vi "Construct Contour SPINE Array (SubVI).vi"(11 "DATA Cluster":T1) -> (0 "Larvae Valid?":bool[](array[boolean]), 1 "Larvae ID":u32[](array[numeric]), 2 "SPINE":cluster{"Array":dbl[], "Array":dbl[]}[](array[cluster]), 3 "Contour":cluster{"Array":i32[], "Array":i32[]}[](array[cluster]), 4 "Frame Valid?":bool)   [LabVIEW 2020]
uses:
  Controls (HOST)/Data to Disk Bundle.ctl
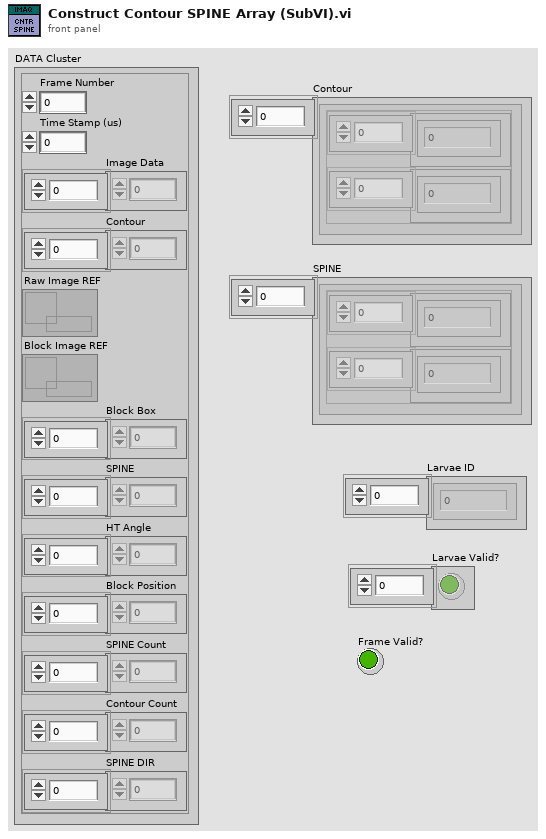
[diagram p1: front panel]
types:
  T1 = typedef "Data to Disk Bundle.ctl" = cluster{"Frame Number":u64, "Time Stamp (us)":u64, "Image Data":u64[], "Contour":u32[], "Raw Image REF":refnum<data-value>, "Block Image REF":refnum<data-value>, "Block Box":u64[], "SPINE":u32[], "HT Angle":u64[], "Block Position":u64[], "SPINE Count":u32[], "Contour Count":u32[], "SPINE DIR":u8[]}
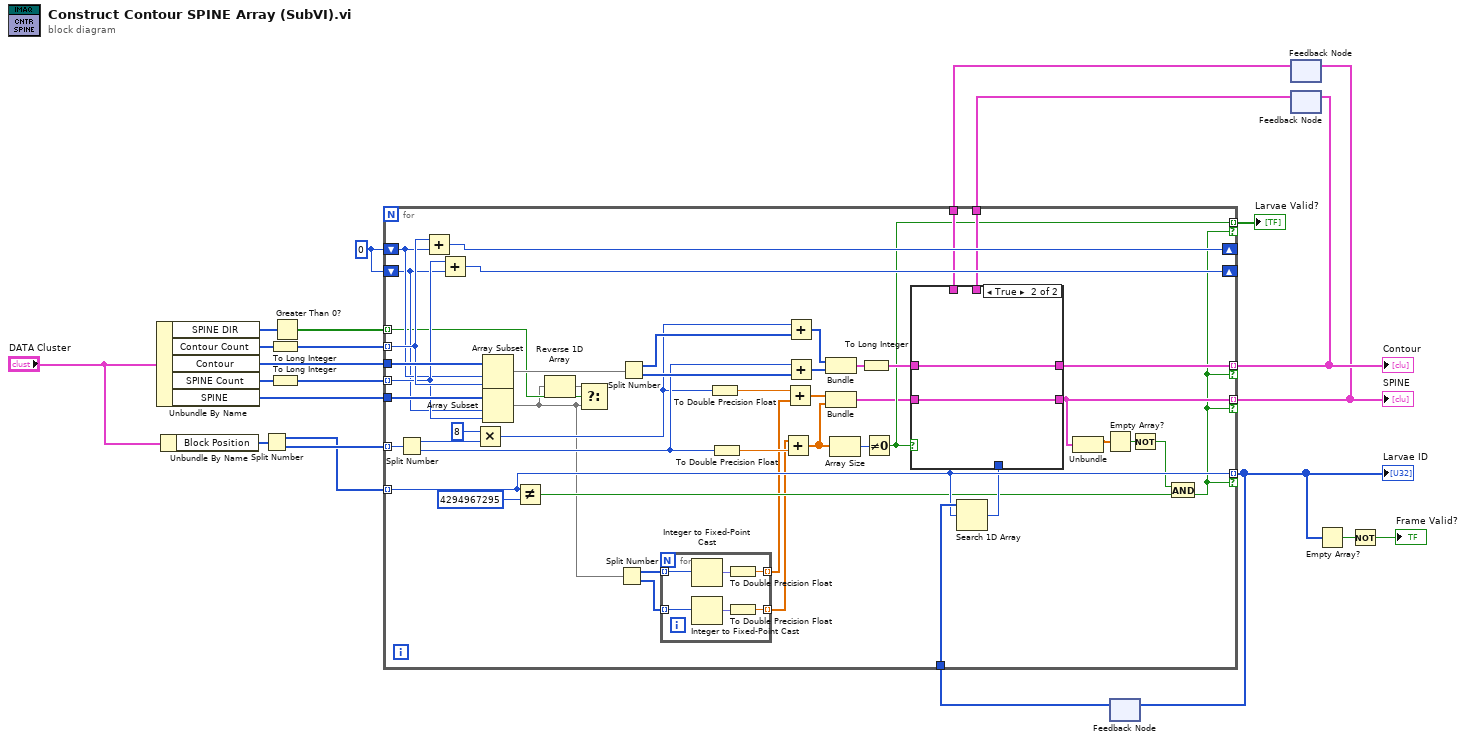
[diagram p0: block diagram]
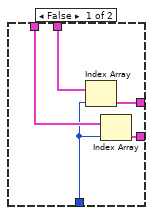
[diagram p2: hidden frame]
diagram:
  w20 = 0 ("Numeric Control")
  n1 = Unbundle By Name("DATA Cluster") -> ("SPINE DIR"=w12:u8[], "Contour Count"=w16:u32[], "Contour"=w17:u32[], "SPINE Count"=w18:u32[], "SPINE"=w19:u32[])
  n2 = Unbundle By Name("DATA Cluster") -> ("Block Position"=w14:u64[])
  n3 = Split Number(x=w14) -> (hi(x)=w10:u32[], lo(x)=w13:u32[])
  n4 = To Long Integer(number=w16) -> (32bit integer=w21:i32[])
  n5 = To Long Integer(number=w18) -> (32bit integer=w22:i32[])
  n6 = Greater Than 0?(x=w12) -> (x > 0?=w11:bool[])
  n7 = feedback #1() -> (w9:u32[])  [unwired: 1 in]
  n8 = feedback #2() -> (w7:cluster{dbl[], dbl[]}[])  [unwired: 1 in]
  n9 = feedback #3() -> (w8:cluster{i32[], i32[]}[])  [unwired: 1 in]
  n10 = for {
    tunnel: w21 -> [w65] mode=indexing
    tunnel: w17 -> [w69]
    tunnel: w22 -> [w64] mode=indexing
    tunnel: w19 -> [w66]
    shift-right: [w68] -> _
    shift-left: w20 -> [w63]
    shift-right: [w67] -> _
    shift-left: w20 -> [w62]
    tunnel: [w41] -> w6 mode=indexing if=w33
    tunnel: [w35] -> w5 mode=indexing if=w33
    tunnel: w13 -> [w57] mode=indexing
    tunnel: w11 -> [w49] mode=indexing
    tunnel: w10 -> [w43] mode=indexing
    tunnel: [w43] -> w2 mode=indexing if=w33
    tunnel: w9 -> [w44]
    tunnel: w8 -> [w40]
    tunnel: w7 -> [w39]
    tunnel: [w37] -> w4 mode=indexing if=w33
    n11 = Split Number(x=w57) -> (hi(x)=w52:u16, lo(x)=w53:u16)
    n12 = Add(x=w65, y=w63) -> (x+y=w68:i32)
    n13 = Add(x=w64, y=w62) -> (x+y=w67:i32)
    n14 = Multiply(x=u16 8, y=w52) -> (x*y=w51:u16)
    n15 = Array Subset(array=w69, index=w63, length=w65) -> (w61:u32[])
    n16 = Array Subset(array=w66, index=w62, length=w64) -> (w23:u32[])
    n17 = Not Equal?(x=w43, y=u32 4294967295) -> (x != y?=w36:bool)
    n18 = Reverse 1D Array(array=w23) -> (reversed array=w48:u32[])
    n19 = Select(t=w48, s=w49, f=w23) -> ()  [unwired: 1 out]
    n20 = Split Number(x=w23) -> (hi(x)=w30:u16[], lo(x)=w29:u16[])
    n21 = Split Number(x=w61) -> (hi(x)=w60:u16[], lo(x)=w59:u16[])
    n22 = for {
      tunnel: w30 -> [w75] mode=indexing
      tunnel: w29 -> [w74] mode=indexing
      tunnel: [w71] -> w26 mode=indexing
      tunnel: [w70] -> w25 mode=indexing
      n23 = Integer to Fixed-Point Cast(integer=w75) -> (fixed-point=w73:fxp<+,16,9>)  [unwired: 1 in]
      n24 = Integer to Fixed-Point Cast(integer=w74) -> (fixed-point=w72:fxp<+,16,9>)  [unwired: 1 in]
      n25 = To Double Precision Float(number=w73) -> (double precision float=w71:dbl)
      n26 = To Double Precision Float(number=w72) -> (double precision float=w70:dbl)
    }
    n27 = To Double Precision Float(number=w51) -> (double precision float=w27:dbl)
    n28 = To Double Precision Float(number=w53) -> (double precision float=w28:dbl)
    n29 = Add(x=w25, y=w28) -> (x+y=w46:dbl[])
    n30 = Add(x=w27, y=w26) -> (x+y=w54:dbl[])
    n31 = Add(x=w51, y=w60) -> (x+y=w56:u16[])
    n32 = Add(x=w53, y=w59) -> (x+y=w55:u16[])
    n33 = Bundle(w56, w55) -> (w58:cluster{u16[], u16[]})  [unwired: 1 in]
    n34 = Bundle(w54, w46) -> (w24:cluster{dbl[], dbl[]})  [unwired: 1 in]
    n35 = Array Size(array=w46) -> (size(s)=w45:i32)
    n36 = To Long Integer(number=w58) -> (32bit integer=w42:cluster{i32[], i32[]})
    n37 = Not Equal To 0?(x=w45) -> (x != 0?=w37:bool)
    n38 = Search 1D Array(1D array=w44, element=w43) -> (index of element=w38:i32)  [unwired: 1 in]
    n39 = case shown="True" w37 {
      tunnel: w42 -> [_ w82]
      tunnel: w24 -> [_ w81]
      tunnel: [w79 w82] -> w41
      tunnel: [w77 w81] -> w35
      tunnel: w40 -> [w80 _]
      tunnel: w39 -> [w78 _]
      tunnel: w38 -> [w76 _]
      frame False {
        n40 = Index Array(array=w80, index=w76) -> (element=w79:cluster{i32[], i32[]})
        n41 = Index Array(array=w78, index=w76) -> (element=w77:cluster{dbl[], dbl[]})
      }
      frame True {
      }
    }
    n42 = Unbundle(w35) -> (w34:dbl[])  [unwired: 1 out]
    n43 = Empty Array?(array=w34) -> (empty?=w32:bool)
    n44 = Not(x=w32) -> (.not. x?=w31:bool)
    n45 = And(x=w31, y=w36) -> (x .and. y?=w33:bool)
  }
  "SPINE" <- w5
  "Contour" <- w6
  "Larvae ID" <- w2
  "Larvae Valid?" <- w4
  n46 = feedback-in #1(w2) -> ()
  n47 = feedback-in #2(w5) -> ()
  n48 = feedback-in #3(w6) -> ()
  n49 = Empty Array?(array=w2) -> (empty?=w3:bool)
  n50 = Not(x=w3) -> (.not. x?=→"Frame Valid?":bool)
